vi "Handle Bool Data.vi"(7 "Source ID":u32, 8 "BoolData":T1, 9 "Sequence":u32, 10 "ChannelService":refnum<class "ChannelService.lvclass">, 11 "Subscription Loop Data in":T2) -> (0 "error out":errorcluster, 3 "Subscription Loop Data":T2)   [LabVIEW 2020, in "Vecto.lvlib" / "RemoteDataService.lvclass"]
uses:
  RemoteDataService.lvclass
  Subscription Loop Data.ctl
  Subscription Group Info.ctl
  Group/Group.lvclass
  SubscribedDataHandler/SubscribedDataHandler.lvclass
  lv-volatus/messages/BoolData/Data.ctl
  ChannelService/ChannelService.lvclass
  <vilib>/Utility/miscctls.llb/LVMapReplaceAction.ctl
  Group/Group.lvclass/Group.ctl
  Group BOOL/Group BOOL.lvclass
  C:/dev/lv20CE/relink/lv-vecto/Vecto/Group/Group.lvclass
  RemoteDataService.lvclass/RemoteDataService.ctl
  Vecto.lvlib
  C:/dev/lv20CE/relink/lv-vecto/Vecto/Group BOOL/Group BOOL.lvclass
  lv-volatus/messages/BoolData/BoolData.lvlib
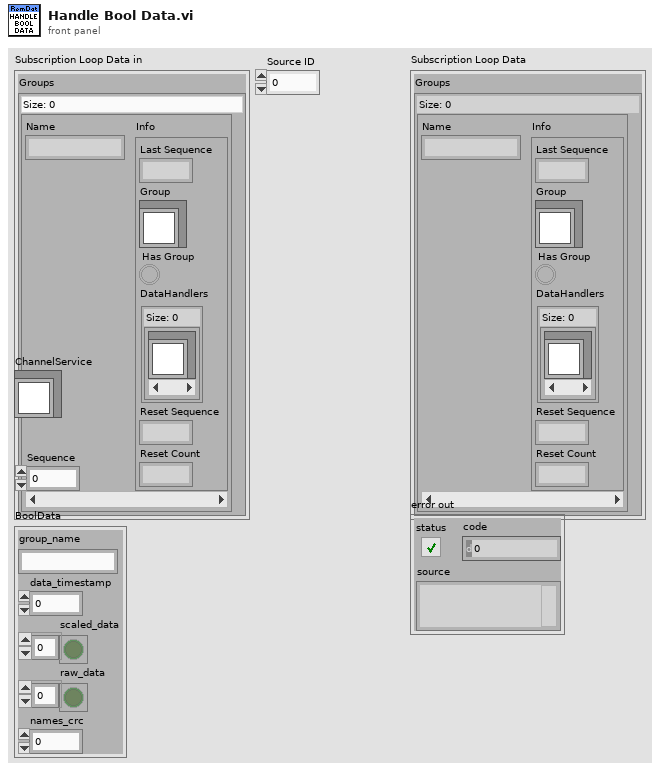
[diagram p1: front panel]
types:
  T1 = typedef "BoolData.lvlib/Data.ctl" = cluster{"group_name":string, "data_timestamp":i64, "scaled_data":bool[], "raw_data":bool[], "names_crc":u32}
  T2 = typedef "Vecto.lvlib/RemoteDataService.lvclass/Subscription Loop Data.ctl" = cluster{"Groups":map{string, T3}}
  T3 = typedef "Vecto.lvlib/RemoteDataService.lvclass/Subscription Group Info.ctl" = cluster{"Last Sequence":u32, "Group":refnum<class "Group.lvclass">, "Has Group":bool, "DataHandlers":set{refnum<class "SubscribedDataHandler.lvclass">}, "Reset Sequence":u32, "Reset Count":u32}
  T4 = typedef "LVMapReplaceAction.ctl" = enum32{"Modify Entry only if found", "Add or Modify Entry", "Delete Entry"}
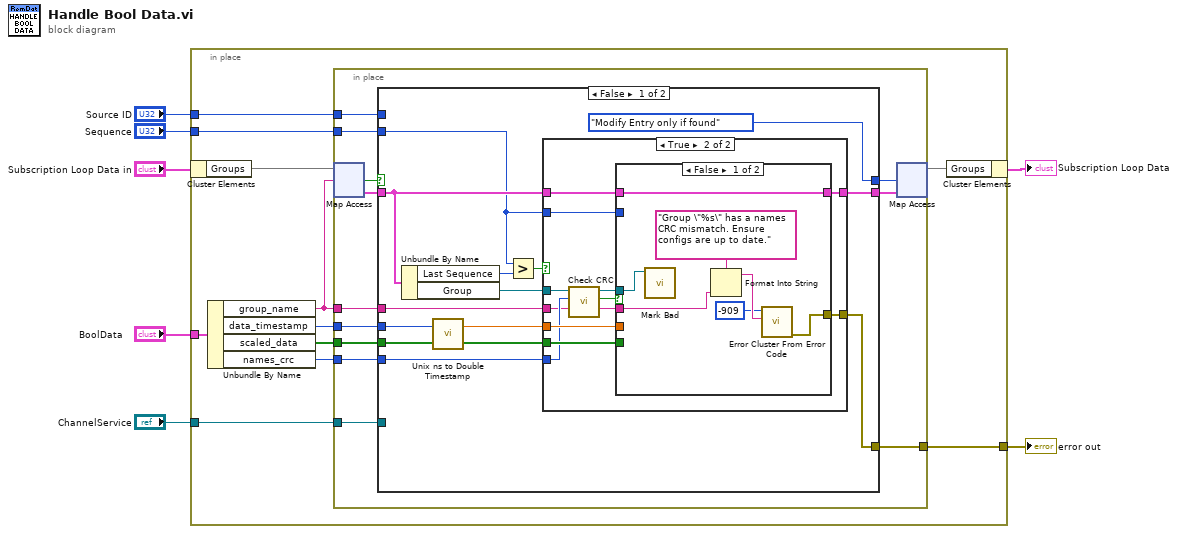
[diagram p0: block diagram]
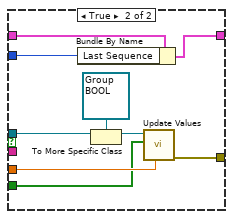
[diagram p3: hidden frame]
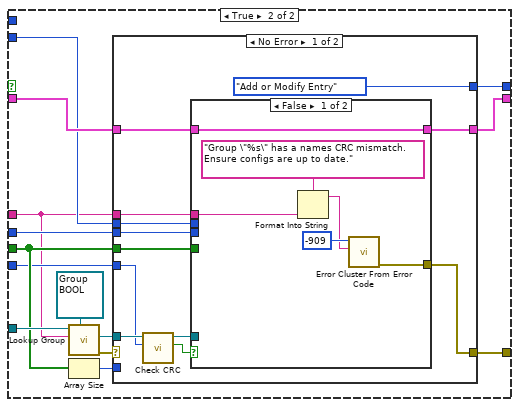
[diagram p4: hidden frame]
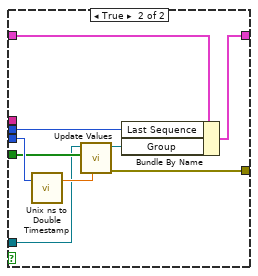
[diagram p5: hidden frame]
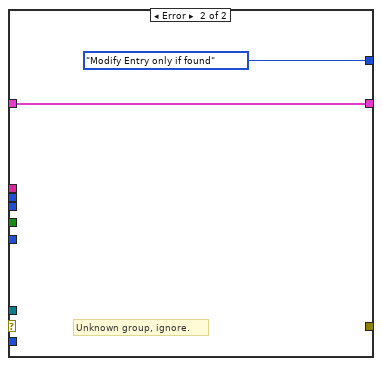
[diagram p6: hidden frame]
diagram:
  n1 = in-place {
    in-place-border: "BoolData" -> [w9]
    in-place-border: "ChannelService" -> [w17]
    in-place-border: "Sequence" -> [w13]
    in-place-border: "Source ID" -> [w12]
    in-place-border: [w10] -> w2
    n2 = in-place-cluster #1("Subscription Loop Data in") -> ("Groups"=w18:map{string, T3})
    n3 = Unbundle By Name(w9) -> ("group_name"=w16:string, "data_timestamp"=w14:i64, "scaled_data"=w15:bool[], "names_crc"=w8:u32)
    n4 = in-place {
      in-place-border: w17 -> [w28]
      in-place-border: w16 -> [w27]
      in-place-border: w15 -> [w26]
      in-place-border: w14 -> [w25]
      in-place-border: w13 -> [w24]
      in-place-border: w12 -> [w23]
      in-place-border: [w21] -> w10
      in-place-border: w8 -> [w19]
      n5 = in-place-map #2(w18, w16) -> (w29:T3, w30:bool)  [unwired: 1 in]
      n6 = case shown="False" w30 {
        tunnel: w29 -> [w38 w81]
        tunnel: w28 -> [_ w85]
        tunnel: w27 -> [w31 w72]
        tunnel: w26 -> [w39 w78]
        tunnel: w25 -> [w40 w79]
        tunnel: w24 -> [w36 w80]
        tunnel: w23 -> [_ _]
        tunnel: [w37 w77] -> w22
        tunnel: [w35 w76] -> w21
        tunnel: [LVMapReplaceAction."Modify Entry only if found" ("action") w75] -> w20
        tunnel: w19 -> [w32 w73]
        frame False {
          n7 = Unbundle By Name(w38) -> ("Last Sequence"=w43:u32, "Group"=w42:refnum<class "Group.lvclass">)
          n8 = call "Unix ns to Double Timestamp.vi"("unix ns"=w40) -> ("Timestamp"=w33:dbl)  [unwired: 2 in]
          n9 = Greater?(x=w36, y=w43) -> (0:w41:bool)
          n10 = case shown="True" w41 {
            tunnel: w42 -> [_ w55]
            tunnel: w33 -> [_ w54]
            tunnel: w39 -> [_ w49]
            tunnel: w38 -> [w44 w53]
            tunnel: [w44 w51] -> w37
            tunnel: w36 -> [_ w52]
            tunnel: [_ w50] -> w35
            tunnel: w32 -> [_ w47]
            tunnel: w31 -> [_ w45]
            frame False {
              # "Older data, ignore"
            }
            frame True {
              n11 = call "Check CRC.vi"("Msg Names CRC"=w47, "Group in"=w55) -> ("CRC Matches"=w46:bool, "Group out"=w48:refnum<class "Group.lvclass">)  [unwired: 8 in]
              n12 = case shown="False" w46 {
                tunnel: w54 -> [_ w71]
                tunnel: w53 -> [w62 w70]
                tunnel: w52 -> [_ w69]
                tunnel: [w62 w68] -> w51
                tunnel: [w57 w67] -> w50
                tunnel: w49 -> [_ w64]
                tunnel: w48 -> [w56 w63]
                tunnel: w45 -> [w58 _]
                frame False {
                  n13 = call "Mark Bad.vi"("Group in"=w56) -> ()  [unwired: 9 in, 2 out]
                  n14 = Format Into String(format string="Group \"%s\" has a names CRC mismatch. Ensure configs are up to date.", w58) -> (resulting string=w61:string)  [unwired: 2 in, 1 out]
                  n15 = call <vilib>:"Error Cluster From Error Code.vi"("error message (\"\")"=w61, "error code (0)"=-909) -> ("error out"=w57:errorcluster)  [unwired: 7 in]
                }
                frame True {
                  n16 = Bundle By Name(cluster=w70, "Last Sequence"=w69) -> (w68:T3)
                  n17 = To More Specific Class(target class=refnum<class "Group BOOL.lvclass"> refnum ("StringGroup in"), reference=w63) -> (specific class reference=w66:refnum<class "Group BOOL.lvclass">)  [unwired: 1 in, 1 out]
                  n18 = call "Update Values.vi"("Timestamp (Now)"=w71, "Values"=w64, "Group BOOL in"=w66) -> ("error out"=w67:errorcluster)  [unwired: 7 in, 1 out]
                }
              }
            }
          }
        }
        frame True {
          n19 = call "Lookup Group.vi"("Group Type (Abstract)"=refnum<class "Group BOOL.lvclass"> refnum ("Vecto.lvlib:StringGroup.lvclass"), "Group Name"=w72, "ChannelService in"=w85) -> ("error out"=w84:errorcluster, "Group"=w83:refnum<class "Group BOOL.lvclass">)  [unwired: 6 in, 1 out]
          n20 = Array Size(array=w78) -> (size(s)=w82:i32)
          n21 = case shown="No Error" w84 {
            tunnel: w83 -> [w91 _]
            tunnel: w82 -> [_ _]
            tunnel: w81 -> [w97 w113]
            tunnel: w80 -> [w96 _]
            tunnel: w79 -> [w92 _]
            tunnel: w78 -> [w89 _]
            tunnel: [w95 w113] -> w77
            tunnel: [w94 _] -> w76
            tunnel: [LVMapReplaceAction."Add or Modify Entry" ("action") LVMapReplaceAction."Modify Entry only if found" ("action")] -> w75
            tunnel: w73 -> [w90 _]
            tunnel: w72 -> [w86 _]
            frame No Error {
              n22 = call "Check CRC.vi"("Msg Names CRC"=w90, "Group in"=w91) -> ("CRC Matches"=w87:bool, "Group out"=w88:refnum<class "Group BOOL.lvclass">)  [unwired: 8 in]
              n23 = case shown="False" w87 {
                tunnel: w97 -> [w103 w112]
                tunnel: w96 -> [_ w111]
                tunnel: [w103 w110] -> w95
                tunnel: [w100 w109] -> w94
                tunnel: w92 -> [_ w106]
                tunnel: w89 -> [_ w105]
                tunnel: w88 -> [_ w104]
                tunnel: w86 -> [w102 _]
                frame False {
                  n24 = Format Into String(format string="Group \"%s\" has a names CRC mismatch. Ensure configs are up to date.", w102) -> (resulting string=w98:string)  [unwired: 2 in, 1 out]
                  n25 = call <vilib>:"Error Cluster From Error Code.vi"("error message (\"\")"=w98, "error code (0)"=-909) -> ("error out"=w100:errorcluster)  [unwired: 7 in]
                }
                frame True {
                  n26 = call "Unix ns to Double Timestamp.vi"("unix ns"=w106) -> ("Timestamp"=w107:dbl)  [unwired: 2 in]
                  n27 = call "Update Values.vi"("Timestamp (Now)"=w107, "Values"=w105, "Group BOOL in"=w104) -> ("error out"=w109:errorcluster, "Group BOOL out"=w108:refnum<class "Group BOOL.lvclass">)  [unwired: 7 in]
                  n28 = Bundle By Name(cluster=w112, "Last Sequence"=w111, "Group"=w108) -> (w110:T3)
                }
              }
            }
            frame Error {
              # "Unknown group, ignore."
            }
          }
        }
      }
      n29 = in-place-map #2(w22, w20) -> (w11:map{string, T3})  [unwired: 2 out]
    }
    n30 = in-place-cluster #1("Groups"=w11) -> (→"Subscription Loop Data":T2)
  }
  "error out" <- w2
